vi "sv_UFF58 Create Channels.vi"(0 "function refnum":refnum<k20>, 1 "real or complex data?":enum16{"Real data", "Complex data"}(ring), 5 "abscissa channel name in":string, 7 "ordinate numerator channel name in":string, 9 "ordinate denominator channel name in":string, 11 "error in (no error)":errorcluster) -> (3 "channel refnums":refnum<k20>[](array[refnum]), 4 "dup function refnum":refnum<k20>, 6 "abscissa channel name out":string, 8 "ordinate numerator channel name out":string, 10 "ordinate denominator channel name out":string, 15 "error out":errorcluster)   [LabVIEW 2017, in "SoundVib_UFF58.lvlib"]
doc: "This VI creates multiple <B>channel refnums</B> depending on the value of <B>real or complex data?</B>. If real, only two channels are created (X and Y). If complex, three channels are created (X, Yreal, and Yimag)."
uses:
  <vilib>/addons/Sound and Vibration/svt_UFF58/SoundVib_UFF58.lvlib
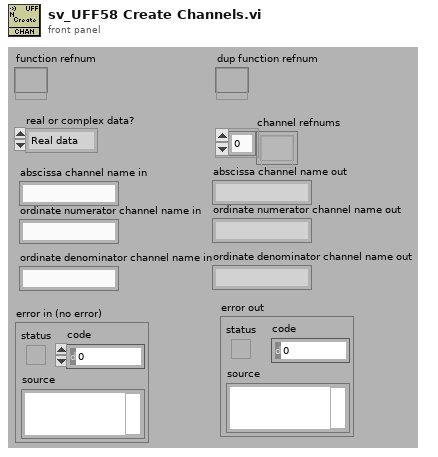
[diagram p1: front panel]
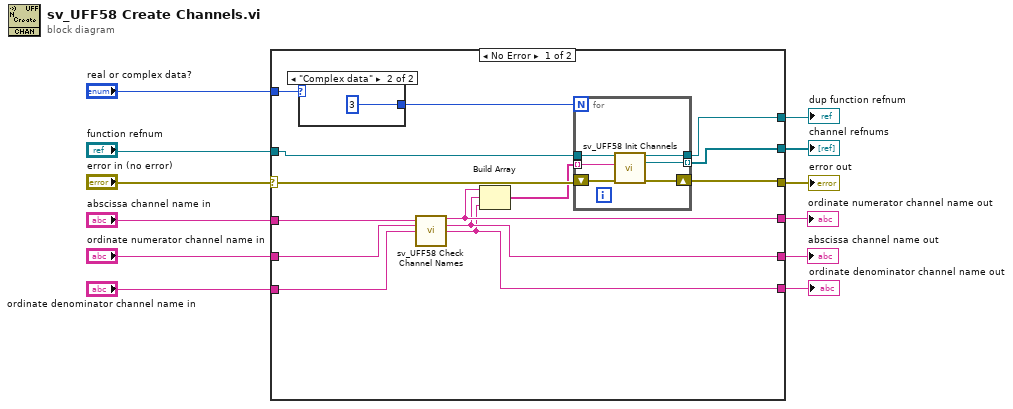
[diagram p0: block diagram]
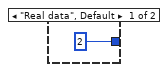
[diagram p2: hidden frame]
diagram:
  n1 = case shown="No Error" "error in (no error)" {
    selector: "error in (no error)" -> [w21 w39]
    tunnel: [w19 w39] -> w12
    tunnel: [w26 w38] -> w5
    tunnel: [w20 _] -> w11
    tunnel: "function refnum" -> [w25 w38]
    tunnel: "real or complex data?" -> [w24 _]
    tunnel: "abscissa channel name in" -> [w22 w37]
    tunnel: "ordinate numerator channel name in" -> [w17 w36]
    tunnel: "ordinate denominator channel name in" -> [w18 w35]
    tunnel: [w15 w37] -> w3
    tunnel: [w14 w36] -> w2
    tunnel: [w13 w35] -> w1
    frame No Error {
      n2 = case shown="\"Complex data\"" w24 {
        tunnel: [2 3] -> w23
        frame "Real data", Default {
        }
        frame "Complex data" {
        }
      }
      n3 = call <vilib>:"sv_UFF58 Check Channel Names.vi"("abscissa channel name"=w22, "ordinate numerator channel name"=w17, "ordinate denominator channel name"=w18) -> ("abscissa channel name out"=w15:string, "ordinate numerator channel name out"=w14:string, "ordinate denominator channel name out"=w13:string)  [unwired: 10 in]
      n4 = Build Array(w15, w14, w13) -> (w16:string[])
      n5 = for {
        N: w23 -> [_]
        tunnel: w25 -> [w34]
        tunnel: [w33] -> w26
        tunnel: [w32] -> w20 mode=indexing
        tunnel: w16 -> [w31] mode=indexing
        shift-right: [w29] -> w19
        shift-left: w21 -> [w30]
        n6 = call <vilib>:"sv_UFF58 Init Channels.vi"("function refnum"=w34, "channel name"=w31, "error in (no error)"=w30) -> ("dup function refnum"=w33:refnum<k20>, "channel refnum"=w32:refnum<k20>, "error out"=w29:errorcluster)  [unwired: 10 in]
      }
    }
    frame Error {
    }
  }
  "error out" <- w12
  "channel refnums" <- w11
  "dup function refnum" <- w5
  "abscissa channel name out" <- w2
  "ordinate numerator channel name out" <- w3
  "ordinate denominator channel name out" <- w1
